vi "Grid Measurements Example - MultipleSpectro.vi"(6 "Internal use":string, 7 "Grid param":T1 {"height (m)" format="%#_6p"; "width (m)" format="%#_6p"; "center Y (m)" format="%#_6p"; "center X (m)" format="%#_6p"}, 8 "Error in (no error)":errorcluster, 9 "Points Y/Index Y":i32, 10 "Points X/Index X":i32, 11 "Method":enum16{"init", "run", "end"}(ring)) -> (0 "Error out":errorcluster)   [LabVIEW 2016]
doc: "Example of a measurement VI to be used in the \"Experiments on a Grid\" tool as external VI.\n\nThis example performs multiple spectroscopy measurement at each point of the grid and saves the data in individual binary files, i.e. the first binary file contains data from the first spectroscopy measurements at each point.\n\n- Nanonis Programming Interface -"
uses:
  Nanonis Prog Interface.lvlib
panel:
  in  "Save Basename":string
  in  "# Spectro. per point":i32=4
  # "Example of a measurement VI to be used in the \"Experiments on a Grid\" tool as external VI.\n\nThis example performs multiple spectroscopy measurement at each point of the grid and saves the data in individual binary files, i.e. the first binary file contains data from the first spectroscopy measurements at each point.\n\nTo use it, set up the bias spectroscopy module to record the desired channels and set all other spectroscopy parameters. Then, set up the experiments on a grid module to use this VI as \"external VI\". On this VI's front panel, adjust the subgrid spacing.\n \n\"Experiments on a Grid\" will first (before starting the measurements) call the external VI with the \"init\" method, passing the grid resolution (Points X, Points Y) and the grid dimensions (Grid param).\nThen, for the measurements, the external VI will be called with the \"run\" method, passing the current X and Y indices (Index X, Index Y).\nAfter the last measurement, the external VI will be called with the \"end\" method.\n\nSee diagram for more information about this example."
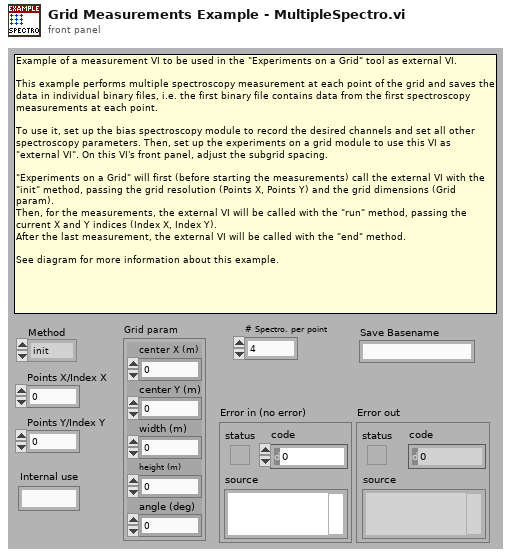
[diagram p1: front panel]
types:
  T1 = cluster{"center X (m)":sgl, "center Y (m)":sgl, "width (m)":sgl, "height (m)":sgl, "angle (deg)":sgl}
  T2 = cluster{"Points X/Index X":i32, "Points Y/Index Y":i32}
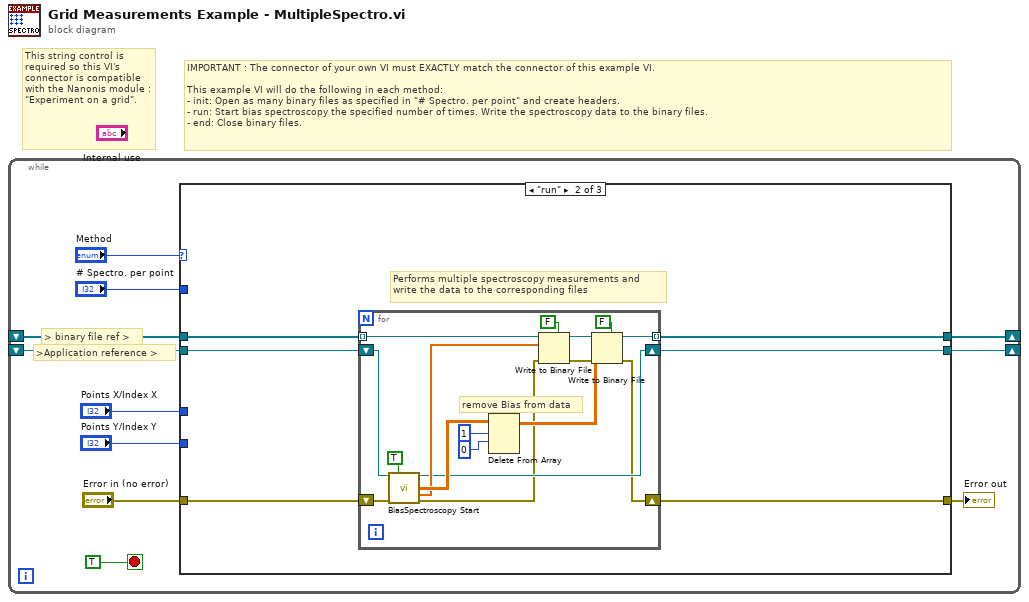
[diagram p0: block diagram]
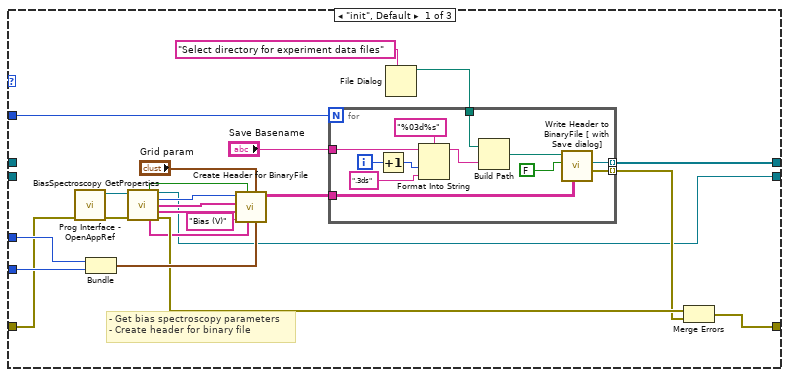
[diagram p2: hidden frame]
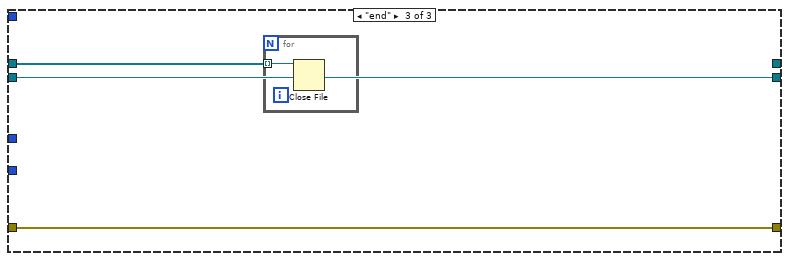
[diagram p3: hidden frame]
diagram:
  # "IMPORTANT : The connector of your own VI must EXACTLY match the connector of this example VI.\n\nThis example VI will do the following in each method:\n- init: Open as many binary files as specified in \"# Spectro. per point\" and create headers.\n- run: Start bias spectroscopy the specified number of times. Write the spectroscopy data to the binary files.\n- end: Close binary files."
  # "This string control is required so this VI's connector is compatible with the Nanonis module : \"Experiment on a grid\"."
  n1 = while {
    shift-right: [w4] -> _
    shift-left: _ -> [w5]
    shift-right: [w2] -> _
    shift-left: _ -> [w1]
    stop <- TRUE stop-if-true
    # ">Application reference >"
    # "> binary file ref >"
    n2 = case shown="\"run\"" "Method" {
      tunnel: "Error in (no error)" -> [w18 w49 w71]
      tunnel: [w28 w52 w71] -> w8
      tunnel: "Points X/Index X" -> [w24 _ _]
      tunnel: "Points Y/Index Y" -> [w23 _ _]
      tunnel: w5 -> [_ w51 w72]
      tunnel: [w27 w50 _] -> w4
      tunnel: "# Spectro. per point" -> [w20 _ _]
      tunnel: [w12 w47 w70] -> w2
      tunnel: w1 -> [_ w48 w70]
      frame "init", Default {
        # "- Get bias spectroscopy parameters\n- Create header for binary file"
        n3 = call <userlib>:"Prog Interface - OpenAppRef.vi"("Error in (no error)"=w18) -> ("Error out"=w17:errorcluster, "Application reference"=w15:refnum<vi>)  [unwired: 5 in]
        n4 = Bundle("Points X/Index X"=w24, "Points Y/Index Y"=w23) -> (w31:T2)  [unwired: 1 in]
        n5 = call <userlib>:"BiasSpectroscopy GetProperties.vi"("Application ref in"=w15, "Error in (no error)"=w17) -> ("Backward sweep"=w32:bool, "Application ref out"=w12:refnum<vi>, "Number of points"=w13:i32, "Channels"=w14:string[], "Parameters"=w30:string[], "Fixed parameters"=w25:string[], "Error out"=w29:errorcluster)  [unwired: 6 in, 1 out]
        n6 = call <userlib>:"Create Header for BinaryFile.vi"("Grid points"=w31, "Grid param"="Grid param", "Fixed parameters"=w25, "Backward sweep"=w32, "Sweep signal"="Bias (V)" ("Sweep Signal"), "Parameters"=w30, "Channels"=w14, "Points per sweep"=w13) -> ("Header (fixed attributes)"=w34:string[][])  [unwired: 3 in]
        n7 = File Dialog(7:"Select directory for experiment data files" ("prompt")) -> (3:w16:path)  [unwired: 6 in, 3 out]
        n8 = for {
          N: w20 -> [_]
          tunnel: w34 -> [w46]
          tunnel: [w45] -> w21 mode=indexing
          tunnel: [w44] -> w27 mode=indexing
          tunnel: "Save Basename" -> [w43]
          tunnel: w16 -> [w35]
          i -> [w41]
          n9 = Increment(x=w41) -> (x+1=w36:i32)
          n10 = Format Into String(format string="%03d%s", initial string=w43, w36, ".3ds" ("input 2")) -> (resulting string=w40:string)  [unwired: 1 in, 1 out]
          n11 = Build Path(base path=w35, name or relative path=w40) -> (appended path=w38:path)
          n12 = call <userlib>:"Write Header to BinaryFile [ with Save dialog].vi"("Fixed Attributes"=w46, "Show Dialog? (T)"=FALSE, "Filename"=w38) -> ("Error out"=w45:errorcluster, "File ref"=w44:refnum<file>)  [unwired: 5 in, 2 out]
        }
        n13 = Merge Errors(w29, w21) -> (w28:errorcluster)
      }
      frame "run" {
        # "Performs multiple spectroscopy measurements and\nwrite the data to the corresponding files"
        n14 = for {
          tunnel: w51 -> [w69] mode=indexing
          tunnel: [w68] -> w50 mode=indexing
          shift-right: [w53] -> w52
          shift-left: w49 -> [w67]
          shift-right: [w57] -> w47
          shift-left: w48 -> [w58]
          # "remove Bias from data"
          n15 = call <userlib>:"BiasSpectroscopy Start.vi"("Application ref in"=w58, "Get data (F)"=TRUE ("Get Data (F)"), "Error in (no error)"=w67) -> ("Application ref out"=w57:refnum<vi>, "Data"=w65:sgl[][], "Parameters"=w59:sgl[], "Error out"=w55:errorcluster)  [unwired: 8 in, 1 out]
          n16 = Delete From Array(array=w65, length=1, index (row)=0 ("index")) -> (array with subset deleted=w64:sgl[][])  [unwired: 1 in, 1 out]
          n17 = Write to Binary File(file (use dialog)=w69, data=w59, error in=w55, 5:FALSE ("prepend array or string size? (T)")) -> (refnum out=w66:refnum<file>, error out=w54:errorcluster)  [unwired: 2 in, 1 out]
          n18 = Write to Binary File(file (use dialog)=w66, data=w64, error in=w54, 5:FALSE ("prepend array or string size? (T)")) -> (refnum out=w68:refnum<file>, error out=w53:errorcluster)  [unwired: 2 in, 1 out]
        }
      }
      frame "end" {
        n19 = for {
          tunnel: w72 -> [w73] mode=indexing
          n20 = Close File(refnum=w73) -> ()  [unwired: 1 in, 2 out]
        }
      }
    }
    "Error out" <- w8
  }
